vi "open_loop_strober.vi"(8 "error in (no error)":errorcluster, 9 "Numeric":dbl, 10 "LED CONTROLS":dbl[][](array[numeric]), 11 "Iteration in":u32) -> (0 "error out":errorcluster, 3 "Iteration out":u32)   [LabVIEW 2013]
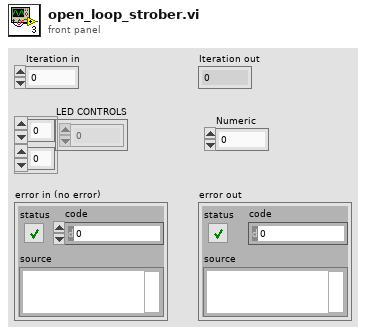
[diagram p1: front panel]
types:
  T1 = enum16{"Set Mode", "Set Normal Current ", "Set Strobe Parameters", "Set Normal Parameters", "Set Strobe Profile "}
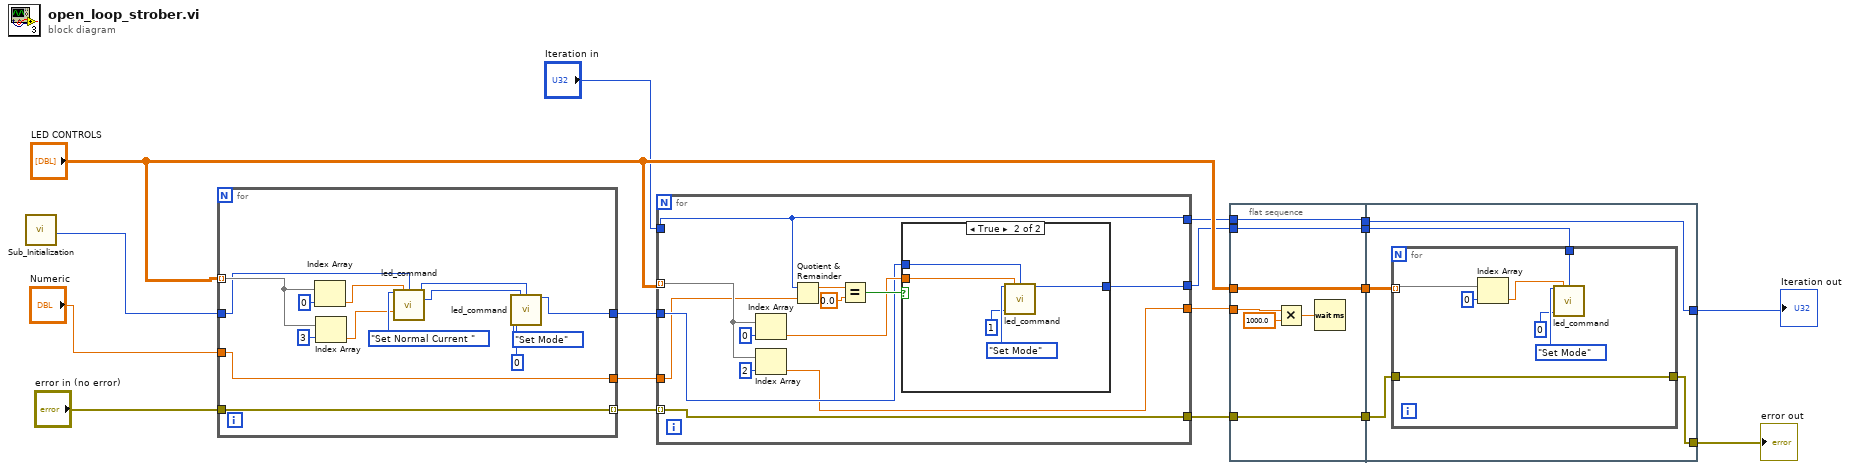
[diagram p0: block diagram]
diagram:
  n1 = call "Sub_Initialization.vi"() -> ("DeviceHandle"=w13:u32)  [unwired: 2 out]
  n2 = for {
    tunnel: "error in (no error)" -> [w32]
    tunnel: [w32] -> w11 mode=indexing
    tunnel: w13 -> [w21]
    tunnel: [w20] -> w12
    tunnel: "LED CONTROLS" -> [w22] mode=indexing
    tunnel: "Numeric" -> [w19]
    tunnel: [w19] -> w1
    n3 = Index Array(array=w22, index=0) -> (element=w29:dbl)
    n4 = Index Array(array=w22, index=3) -> (element=w27:dbl)
    n5 = call "led_command.vi"("COMMAND"=T1."Set Normal Current ", "Channel"=w29, "Device Handle"=w21, "Iset"=w27) -> ("Device Handle Out"=w24:u32, "Channel Out"=w25:i32)  [unwired: 8 in, 2 out]
    n6 = call "led_command.vi"("COMMAND"=T1."Set Mode", "Channel"=w25, "Device Handle"=w24, "Mode"=u32 0) -> ("Device Handle Out"=w20:u32)  [unwired: 8 in, 3 out]
  }
  n7 = for {
    tunnel: "Iteration in" -> [w36]
    tunnel: "LED CONTROLS" -> [w34] mode=indexing
    tunnel: w12 -> [w39]
    tunnel: [w38] -> w4
    tunnel: [w37] -> w5
    tunnel: [w36] -> w6
    tunnel: [w35] -> w8
    tunnel: w11 -> [w35] mode=indexing
    tunnel: w1 -> [w33]
    n8 = Index Array(array=w34, index=0) -> (element=w40:dbl)
    n9 = Index Array(array=w34, index=2) -> (element=w38:dbl)
    n10 = Quotient & Remainder(x=w36, y=w33) -> (x-y*floor(x/y)=w45:dbl)  [unwired: 1 out]
    n11 = Equal?(x=w45, y=0.0) -> (x = y?=w43:bool)
    n12 = case shown="True" w43 {
      tunnel: w40 -> [_ w49]
      tunnel: w39 -> [w46 w48]
      tunnel: [w46 w47] -> w37
      frame False {
      }
      frame True {
        n13 = call "led_command.vi"("COMMAND"=T1."Set Mode", "Channel"=w49, "Device Handle"=w48, "Mode"=u32 1) -> ("Device Handle Out"=w47:u32)  [unwired: 8 in, 3 out]
      }
    }
  }
  n14 = flat-sequence {
    tunnel: "LED CONTROLS" -> [w58]
    tunnel: w4 -> [w57]
    tunnel: [w58] -> w18
    tunnel: w5 -> [w54]
    tunnel: [w54] -> w17
    tunnel: w6 -> [w53]
    tunnel: [w53] -> w16
    tunnel: w8 -> [w52]
    tunnel: [w52] -> w15
    tunnel: w18 -> [w63]
    tunnel: w17 -> [w62]
    tunnel: w16 -> [w61]
    tunnel: [w61] -> w7
    tunnel: w15 -> [w60]
    tunnel: [w59] -> w9
    frame #0 {
      n15 = Multiply(x=w57, y=1000.0) -> (x*y=w56:dbl)
      n16 = Wait (ms)(milliseconds to wait=w56) -> ()  [unwired: 1 out]
    }
    frame #1 {
      n17 = for {
        tunnel: w63 -> [w64] mode=indexing
        tunnel: w62 -> [w67]
        tunnel: w60 -> [w65]
        tunnel: [w65] -> w59
        n18 = Index Array(array=w64, index=0) -> (element=w66:dbl)
        n19 = call "led_command.vi"("COMMAND"=T1."Set Mode", "Channel"=w66, "Device Handle"=w67, "Mode"=u32 0) -> ()  [unwired: 8 in, 4 out]
      }
    }
  }
  "error out" <- w9
  "Iteration out" <- w7
